vi "Create Line by Two Points.vi"(8 "error in (no error)":errorcluster caption="错误输入（无错误）", 10 "EndPointB":refnum<class "Point.lvclass">, 11 "EndPointA":refnum<class "Point.lvclass">) -> (0 "error out":errorcluster caption="错误输出")   [LabVIEW 2011, in "Line.lvclass"]
uses:
  Line.lvclass
  Point/Point.lvclass
panel:
  out "PerToX":bool
  out "b":dbl
  out "K":dbl
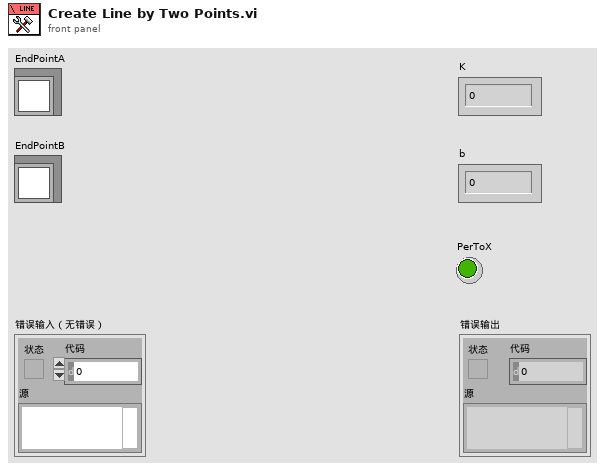
[diagram p1: front panel]
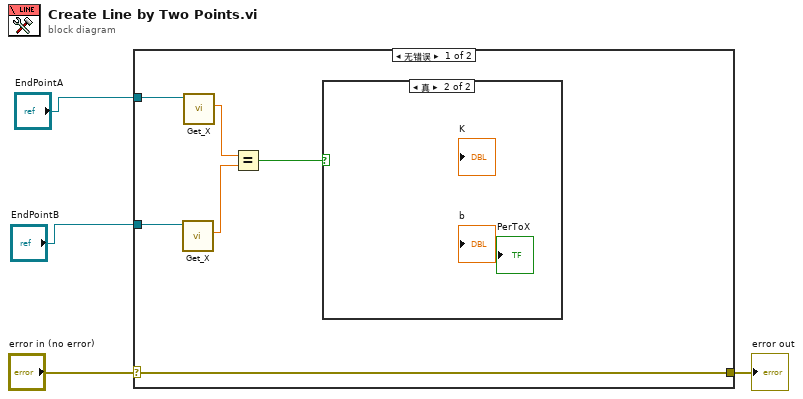
[diagram p0: block diagram]
diagram:
  n1 = case shown="无错误" "error in (no error)" {
    selector: "error in (no error)" -> [w10 w11]
    tunnel: [w10 w11] -> w3
    tunnel: "EndPointA" -> [w9 _]
    tunnel: "EndPointB" -> [w8 _]
    frame No Error {
      n2 = call "Get_X.vi"("Point输入"=w8) -> ("X"=w6:dbl)  [unwired: 8 in, 2 out]
      n3 = call "Get_X.vi"("Point输入"=w9) -> ("X"=w7:dbl)  [unwired: 8 in, 2 out]
      n4 = Equal?(x=w7, y=w6) -> (x = y?=w5:bool)
      n5 = case shown="真" w5 {
        frame False {
        }
        frame True {
        }
      }
    }
    frame Error {
    }
  }
  "error out" <- w3
